vi "Test Detect Tags.vi"(11 "Test Case In":refnum<class "02_FeatureDetectionAprilTag.lvclass">) -> (0 "error out":errorcluster, 3 "Test Case Out":refnum<class "02_FeatureDetectionAprilTag.lvclass">)   [LabVIEW 2020, in "test.lvlib" / "02_FeatureDetectionAprilTag.lvclass"]
uses:
  02_FeatureDetectionAprilTag.lvclass
  C:/Program Files (x86)/National Instruments/LabVIEW 2026/vi.lib/Astemes/LUnit/Test Case.lvclass
  feature_detection/Apriltag Detector/Detector Settings.ctl
  02_FeatureDetectionAprilTag.lvclass/02_FeatureDetectionAprilTag.ctl
  feature_detection/Apriltag Detector/AprilTag Detector.lvclass/AprilTag Detector.ctl
  <vilib>/Astemes/LUnit/Test Case.lvclass/Test Case.ctl
  feature_detection/AprilTag ID List (Tag16h5).vi
  feature_detection/Apriltag Detector/Create (Tag16h5).vi
  feature_detection/AprilTag ID List (Tag25h9).vi
  feature_detection/Apriltag Detector/Create (Tag25h9).vi
  feature_detection/AprilTag ID List (Tag36h11).vi
  feature_detection/Apriltag Detector/Create (Tag36h11).vi
  feature_detection/AprilTag ID List (TagCircle21h7).vi
  feature_detection/Apriltag Detector/Create (Circle21h7).vi
  feature_detection/AprilTag ID List (TagCircle49h12).vi
  feature_detection/Apriltag Detector/Create  (Circle 49h12).vi
  feature_detection/AprilTag ID List (TagCustom48h12).vi
  feature_detection/Apriltag Detector/Create (TagCustom48h12).vi
  feature_detection/AprilTag ID List (TagStandard41h12).vi
  feature_detection/Apriltag Detector/Create (TagStandard41h12).vi
  feature_detection/AprilTag ID List (TagStandard52h13).vi
  feature_detection/Apriltag Detector/Create (TagStandard52h13).vi
  image/New Image (Greyscale Array).vi
  4993e8ee-a06a-463a-9684-69129f64d5ce.vi
  <vilib>/Astemes/LUnit/Core/LUnit Test Case/Private/Append Pass Result.vi
  <vilib>/Astemes/LUnit/Core/LUnit Test Case/Private/Append Fail Result.vi
  4993e8ee-a06a-463a-9684-69129f64d5ce.vi/9c5d11cd-9439-4240-a1ee-d9baace9c924.vi
  <vilib>/Astemes/LUnit/Core/LUnit Test Case/Private/Run In UI.vi
  <vilib>/Utility/error.llb/Clear Errors.vi
  feature_detection/AprilTag16h5Codes.vi
  feature_detection/Apriltag Detector/CreateDetector.vi
  feature_detection/Generate Apriltag Image Data (Tag16h5).vi
  feature_detection/AprilTag36h11Codes.vi
  feature_detection/Generate Apriltag Image Data (Tag25h9).vi
  feature_detection/Generate Apriltag Image Data (Tag36h11).vi
  feature_detection/AprilTagCircle21h7Codes.vi
  feature_detection/Generate Apriltag Image Data (TagCircle21h7).vi
  feature_detection/AprilTagCircle49h12Codes.vi
  feature_detection/Generate Apriltag Image Data (TagCircle49h12).vi
  feature_detection/AprilTagCustom48h12Codes.vi
  feature_detection/Generate Apriltag Image Data (TagCustom48h12).vi
  feature_detection/AprilTagStandard41h12Codes.vi
  feature_detection/Generate Apriltag Image Data (TagStandard41h12).vi
  feature_detection/AprilTagStandard52h13Codes.vi
  feature_detection/Generate Apriltag Image Data (TagStandard52h13).vi
  <vilib>/Utility/error.llb/Error Cluster From Error Code.vi
  feature_detection/Apriltag Detector/AprilTag Detector.lvclass
  feature_detection/feature_detection.lvlib
  image/image.lvlib
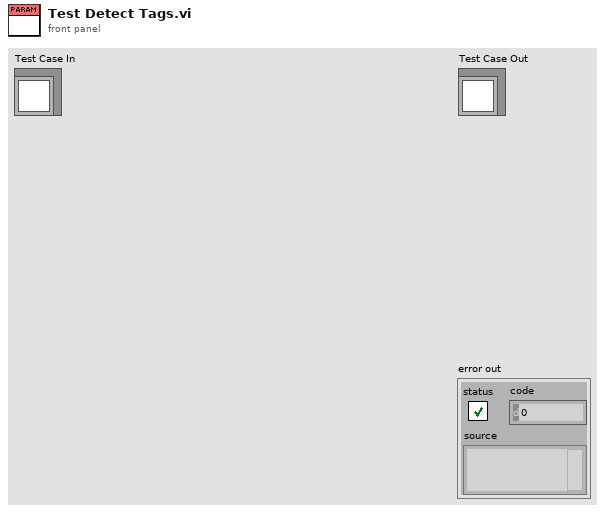
[diagram p1: front panel]
types:
  T1 = typedef "feature_detection.lvlib/AprilTag Detector.lvclass/Detector Settings.ctl" = cluster{"Refine Edges (Default: True)":bool, "Threads (Default: 1)":u8, "Decimate (Default: 1)":sgl, "Blur (Default: 0)":sgl, "Bits (Default: 2)":u8}
  T2 = typedef "common.lvlib/Quad Corners.ctl" = cluster{"Bottom Left":T3, "Bottom Right":T3, "Top Right":T3, "Top Left":T3}
  T3 = typedef "common.lvlib/Image Point (Float).ctl" = cluster{"x":dbl, "y":dbl}
  T4 = enum8{"tag16h5", "tag25h9", "tag36h11", "tagCircle21h7", "tagCircle49h12", "tagCustom48h12", "tagStandard41h12", "tagStandard52h13"}
  T5 = cluster{cluster{"x":i32, "y":i32}, cluster{"x":i32, "y":i32}, cluster{"x":i32, "y":i32}, cluster{"x":i32, "y":i32}}
  T6 = typedef "image.lvlib/Greyscale Image.ctl" = refnum<data-value>
  T7 = typedef "feature_detection.lvlib/AprilTag Detector.lvclass/Detection.ctl" = cluster{"ID":i32, "Hamming":i32, "Decision Margin":sgl, "Centre":T3, "Corners":T2}
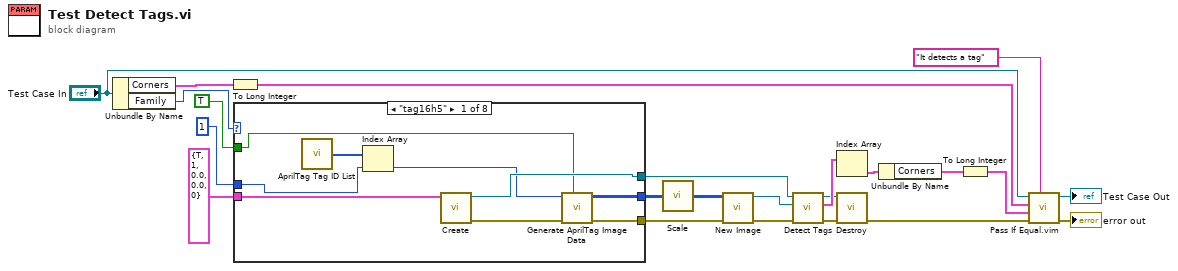
[diagram p0: block diagram]
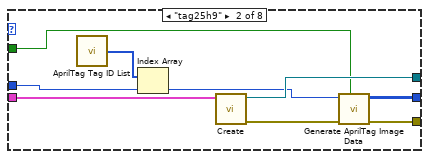
[diagram p2: hidden frame]
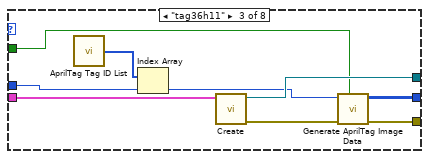
[diagram p3: hidden frame]
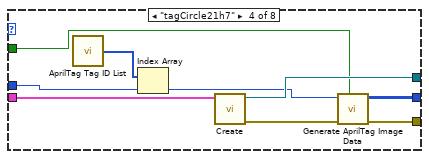
[diagram p4: hidden frame]
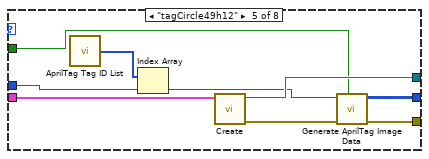
[diagram p5: hidden frame]
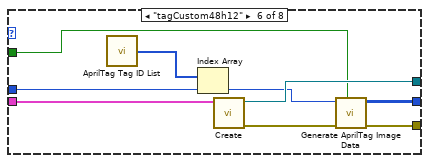
[diagram p6: hidden frame]
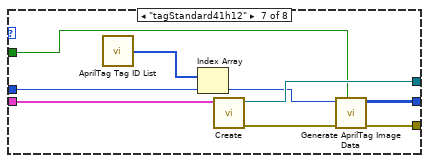
[diagram p7: hidden frame]
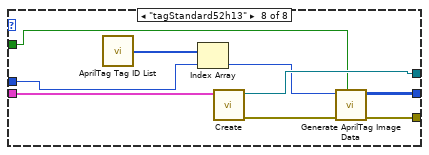
[diagram p8: hidden frame]
diagram:
  n1 = Unbundle By Name("Test Case In") -> ("Corners"=w7:T2, "Family"=w4:T4)
  n2 = To Long Integer(number=w7) -> (32bit integer=w2:T5)
  n3 = case shown="\"tag16h5\"" w4 {
    tunnel: [w32 w34 w43 w59 w68 w77 w86 w95] -> w20
    tunnel: [w31 w41 w50 w58 w67 w76 w85 w94] -> w13
    tunnel: [w27 w37 w46 w54 w63 w72 w81 w90] -> w19
    tunnel: T1 {"Refine Edges (Default: True)"=TRUE, "Threads (Default: 1)"=1, "Decimate (Default: 1)"=0.0, "Blur (Default: 0)"=0.0, "Bits (Default: 2)"=0} ("Detector Settings") -> [w26 w36 w45 w53 w62 w71 w80 w89]
    tunnel: 1 ("index") -> [w25 w35 w44 w52 w61 w70 w79 w88]
    tunnel: TRUE ("Add Border (Default: False)") -> [w24 w33 w42 w51 w60 w69 w78 w87]
    frame "tag16h5" {
      n4 = call-poly "AprilTag Tag ID List.vi"() -> ("Tag IDs"=w30:i32[])
      n5 = Index Array(array=w30, index=w25) -> (element=w29:i32)
      n6 = call-poly "Create.vi"("Detector Settings"=w26) -> ("error out"=w28:errorcluster, "Apriltag Detector"=w31:refnum<class "AprilTag Detector.lvclass">)  [unwired: 9 in]
      n7 = call-poly "Generate AprilTag Image Data.vi"("Add Border (Default: False)"=w24, "error in (no error)"=w28, "ID"=w29) -> ("error out"=w27:errorcluster, "Tag Image Data"=w32:u8[][])  [unwired: 7 in]
    }
    frame "tag25h9" {
      n8 = call-poly "AprilTag Tag ID List.vi"() -> ("Tag IDs"=w40:i32[])
      n9 = Index Array(array=w40, index=w35) -> (element=w39:i32)
      n10 = call-poly "Create.vi"("Detector Settings"=w36) -> ("error out"=w38:errorcluster, "Apriltag Detector"=w41:refnum<class "AprilTag Detector.lvclass">)  [unwired: 9 in]
      n11 = call-poly "Generate AprilTag Image Data.vi"("Add Border (Default: False)"=w33, "error in (no error)"=w38, "ID"=w39) -> ("error out"=w37:errorcluster, "Tag Image Data"=w34:u8[][])  [unwired: 7 in]
    }
    frame "tag36h11" {
      n12 = call-poly "AprilTag Tag ID List.vi"() -> ("Tag IDs"=w49:i32[])
      n13 = Index Array(array=w49, index=w44) -> (element=w48:i32)
      n14 = call-poly "Create.vi"("Detector Settings"=w45) -> ("error out"=w47:errorcluster, "Apriltag Detector"=w50:refnum<class "AprilTag Detector.lvclass">)  [unwired: 9 in]
      n15 = call-poly "Generate AprilTag Image Data.vi"("Add Border (Default: False)"=w42, "error in (no error)"=w47, "ID"=w48) -> ("error out"=w46:errorcluster, "Tag Image Data"=w43:u8[][])  [unwired: 7 in]
    }
    frame "tagCircle21h7" {
      n16 = call-poly "AprilTag Tag ID List.vi"() -> ("Tag IDs"=w57:i32[])
      n17 = Index Array(array=w57, index=w52) -> (element=w56:i32)
      n18 = call-poly "Create.vi"("Detector Settings"=w53) -> ("error out"=w55:errorcluster, "Apriltag Detector"=w58:refnum<class "AprilTag Detector.lvclass">)  [unwired: 9 in]
      n19 = call-poly "Generate AprilTag Image Data.vi"("Add Border (Default: False)"=w51, "error in (no error)"=w55, "ID"=w56) -> ("error out"=w54:errorcluster, "Tag Image Data"=w59:u8[][])  [unwired: 6 in, 1 out]
    }
    frame "tagCircle49h12" {
      n20 = call-poly "AprilTag Tag ID List.vi"() -> ("Tag IDs"=w66:i32[])
      n21 = Index Array(array=w66, index=w61) -> (element=w65:i32)
      n22 = call-poly "Create.vi"("Detector Settings"=w62) -> ("error out"=w64:errorcluster, "Apriltag Detector"=w67:refnum<class "AprilTag Detector.lvclass">)  [unwired: 9 in]
      n23 = call-poly "Generate AprilTag Image Data.vi"("Add Border (Default: False)"=w60, "error in (no error)"=w64, "ID"=w65) -> ("error out"=w63:errorcluster, "Tag Image Data"=w68:u8[][])  [unwired: 6 in, 1 out]
    }
    frame "tagCustom48h12" {
      n24 = call-poly "AprilTag Tag ID List.vi"() -> ("Tag IDs"=w75:i32[])
      n25 = Index Array(array=w75, index=w70) -> (element=w74:i32)
      n26 = call-poly "Create.vi"("Detector Settings"=w71) -> ("error out"=w73:errorcluster, "Apriltag Detector"=w76:refnum<class "AprilTag Detector.lvclass">)  [unwired: 9 in]
      n27 = call-poly "Generate AprilTag Image Data.vi"("Add Border (Default: False)"=w69, "error in (no error)"=w73, "ID"=w74) -> ("error out"=w72:errorcluster, "Tag Image Data"=w77:u8[][])  [unwired: 6 in, 1 out]
    }
    frame "tagStandard41h12" {
      n28 = call-poly "AprilTag Tag ID List.vi"() -> ("Tag IDs"=w84:i32[])
      n29 = Index Array(array=w84, index=w79) -> (element=w83:i32)
      n30 = call-poly "Create.vi"("Detector Settings"=w80) -> ("error out"=w82:errorcluster, "Apriltag Detector"=w85:refnum<class "AprilTag Detector.lvclass">)  [unwired: 9 in]
      n31 = call-poly "Generate AprilTag Image Data.vi"("Add Border (Default: False)"=w78, "error in (no error)"=w82, "ID"=w83) -> ("error out"=w81:errorcluster, "Tag Image Data"=w86:u8[][])  [unwired: 7 in]
    }
    frame "tagStandard52h13" {
      n32 = call-poly "AprilTag Tag ID List.vi"() -> ("Tag IDs"=w93:i32[])
      n33 = Index Array(array=w93, index=w88) -> (element=w92:i32)
      n34 = call-poly "Create.vi"("Detector Settings"=w89) -> ("error out"=w91:errorcluster, "Apriltag Detector"=w94:refnum<class "AprilTag Detector.lvclass">)  [unwired: 9 in]
      n35 = call-poly "Generate AprilTag Image Data.vi"("Add Border (Default: False)"=w87, "error in (no error)"=w91, "ID"=w92) -> ("error out"=w90:errorcluster, "Tag Image Data"=w95:u8[][])  [unwired: 7 in]
    }
  }
  n36 = call "Scale.vi"("Tag Pixel Array in"=w20) -> ("Tag Pixel Array out"=w5:u8[][])
  n37 = call-poly "New Image.vi"("error in (no error)"=w19, "U8 Greyscale Data"=w5) -> ("error out"=w17:errorcluster, "Greyscale Image"=w8:T6)  [unwired: 8 in]
  n38 = call "Detect Tags.vi"("error in (no error)"=w17, "Greyscale Image in"=w8, "Apriltag Detector in"=w13) -> ("error out"=w16:errorcluster, "Detections"=w15:T7[], "Apriltag Detector"=w10:refnum<class "AprilTag Detector.lvclass">)  [unwired: 4 in, 2 out]
  n39 = Index Array(array=w15) -> (element=w14:T7)  [unwired: 1 in]
  n40 = call "Destroy.vi"("error in (no error)"=w16, "Apriltag Detector in"=w10) -> ("error out"=w12:errorcluster)  [unwired: 9 in]
  n41 = Unbundle By Name(w14) -> ("Corners"=w6:T2)
  n42 = To Long Integer(number=w6) -> (32bit integer=w3:T5)
  n43 = call "Pass If Equal.vim"("Description"="It detects a tag", "error in (no error)"=w12, "Actual"=w3, "Expected"=w2, "LUnit Test Case In"="Test Case In") -> ("error out"=→"error out":errorcluster, "LUnit Test Case Out"=→"Test Case Out":refnum<class "02_FeatureDetectionAprilTag.lvclass">)  [unwired: 5 in]
